vi "Update.vi"(8 "error in (no error)":errorcluster, 10 "Message in":refnum<class "UpdateMessage.lvclass">, 11 "BMC in":refnum<class "BMC.lvclass">) -> (0 "error out":errorcluster, 3 "BMC out":refnum<class "BMC.lvclass">)   [LabVIEW 2012, in "BMC.lvclass"]
doc: "The update method processes the command 'update'. \n\nThe command 'update' is used for receiving new values to be set to the private data of the class. This could be seen as a public set method for setting new parameters to the private class data."
uses:
  BMC.lvclass
  <vilib>/Distrio/Murmex/UpdateMessage/UpdateMessage.lvclass
  BMC.lvclass/BMC.ctl
  <vilib>/Distrio/Murmex/Murmex/Murmex.lvclass
panel:
  # "This method is called when the UPDATE\ntrigger is sent. \n\nOverride this method when your component needs to\nrespond to this trigger. \n\nCall parent for proper implementation"
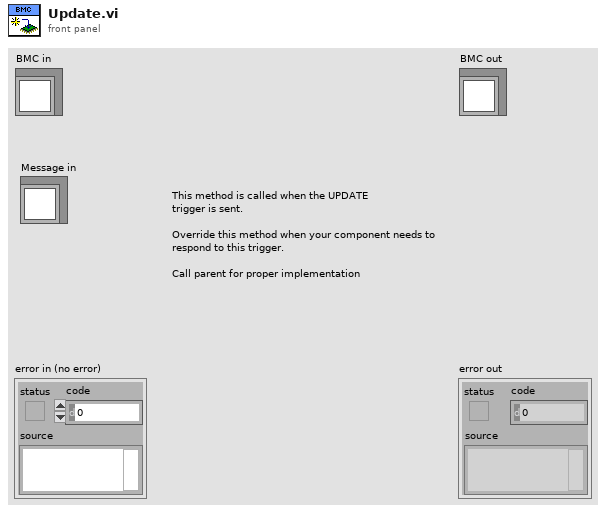
[diagram p1: front panel]
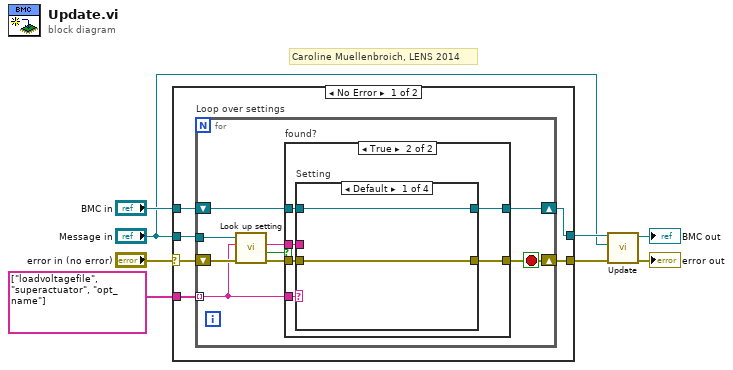
[diagram p0: block diagram]
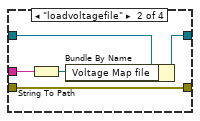
[diagram p3: hidden frame]
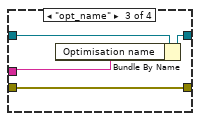
[diagram p4: hidden frame]
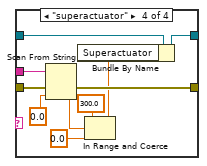
[diagram p5: hidden frame]
diagram:
  # "Caroline Muellenbroich, LENS 2014"
  n1 = case shown="No Error" "error in (no error)" {
    selector: "error in (no error)" -> [w10 w53]
    tunnel: string[] ["loadvoltagefile", "superactuator", "opt_name"] ("key chains") -> [w14 _]
    tunnel: "Message in" -> [w9 _]
    tunnel: "BMC in" -> [w13 w54]
    tunnel: [w11 w53] -> w5
    tunnel: [w12 w54] -> w3
    frame No Error {
      n2 = for "Loop over settings" {
        shift-right: [w15] -> w11
        shift-left: w10 -> [w23]
        tunnel: w14 -> [w17] mode=indexing
        tunnel: w9 -> [w22]
        shift-right: [w16] -> w12
        shift-left: w13 -> [w20]
        stop <- w15 stop-if-true
        n3 = call <vilib>:"Look up setting.vi"("error in (no error)"=w23, "tag name"=w17, "UpdateMessage in"=w22) -> ("error out"=w18:errorcluster, "found?"=w21:bool, "value"=w19:string)  [unwired: 5 in, 1 out]
        n4 = case "found?" shown="True" w21 {
          tunnel: w20 -> [w25 w29]
          tunnel: w19 -> [_ w30]
          tunnel: w18 -> [w24 w28]
          tunnel: w17 -> [_ w31]
          tunnel: [w25 w27] -> w16
          tunnel: [w24 w26] -> w15
          frame False {
          }
          frame True {
            n5 = case "Setting" shown="Default" w31 {
              tunnel: w30 -> [_ w35 w40 w51]
              tunnel: w29 -> [w33 w38 w41 w50]
              tunnel: w28 -> [w32 w36 w39 w52]
              tunnel: [w33 w37 w42 w49] -> w27
              tunnel: [w32 w36 w39 w48] -> w26
              frame Default {
              }
              frame "loadvoltagefile" {
                n6 = String To Path(string=w35) -> (path=w34:path)
                n7 = Bundle By Name(cluster=w38, "Voltage Map file"=w34) -> (w37:refnum<class "BMC.lvclass">)
              }
              frame "opt_name" {
                n8 = Bundle By Name(cluster=w41, "Optimisation name"=w40) -> (w42:refnum<class "BMC.lvclass">)
              }
              frame "superactuator" {
                n9 = Scan From String(input string=w51, error in=w52, default 1=0.0 ("settings.Superactuator")) -> (error out=w48:errorcluster, output 1=w44:dbl)  [unwired: 2 in, 2 out]
                n10 = In Range and Coerce(upper limit=300.0, x=w44, lower limit=0.0) -> (coerced(x)=w43:dbl)  [unwired: 1 out]
                n11 = Bundle By Name(cluster=w50, "Superactuator"=w43) -> (w49:refnum<class "BMC.lvclass">)
              }
            }
          }
        }
      }
    }
    frame Error {
    }
  }
  n12 = call-parent "Update.vi"("error in (no error)"=w5, "Message in"="Message in", "Murmex in"=w3) -> ("error out"=→"error out":errorcluster, "Murmex out"=→"BMC out":refnum<class "BMC.lvclass">)  [unwired: 7 in]
